vi "WPI_UtilitiesTestComplete.vi"(9 "Name":string, 11 "Boolean":bool) -> ()   [LabVIEW 2017]
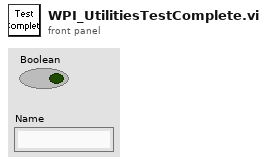
[diagram p1: front panel]
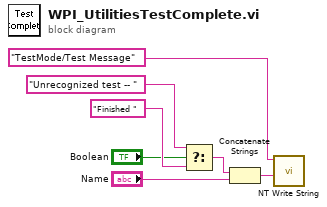
[diagram p0: block diagram]
diagram:
  n1 = Select(t="Unrecognized test -- " ("Name"), s="Boolean", f="Finished " ("Name")) -> (s? t:f=w3:string)
  n2 = Concatenate Strings(w3, "Name") -> (w2:string)
  n3 = call <vilib>:"NT Write String.vi"("String"=w2, "Name"="TestMode/Test Message") -> ()  [unwired: 9 in, 1 out]
